vi "Write Test.vi"() -> ()   [LabVIEW 2020]
uses:
  <vilib>/Platform/TimedLoop/XDataNode/timing_clust.ctl
  <vilib>/Platform/TimedLoop/XDataNode/nitl_modes.ctl
  <vilib>/Platform/TimedLoop/XDataNode/wakeup.ctl
  <vilib>/platform/TimedLoop/XDataNode/XDataNode.xnode
  <vilib>/measure/NI_MABase.lvlib
  <vilib>/Platform/TimedLoop/XDataNode/XDNodeRunTimeDep.lvlib
panel:
  out "x-y":dbl
  out "Array":i32[](array[numeric])
  out "x+y":i32[](array[numeric])
  in  "stop":bool
  out "Storage Time":dbl format="%<%H:%M:%S%3u>t"
  in  "Count":i32
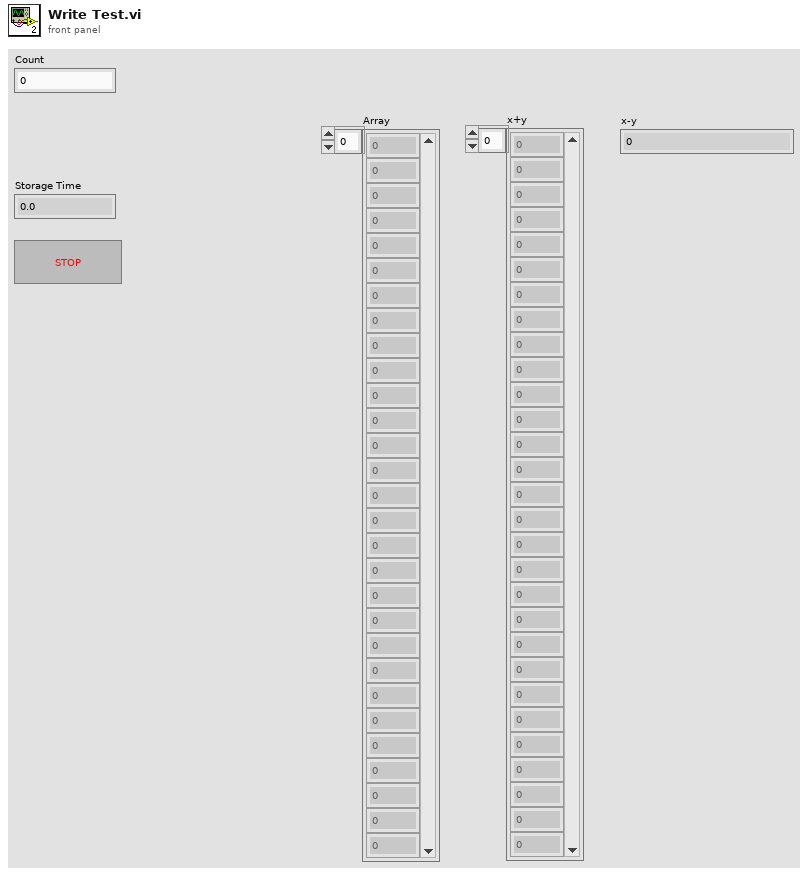
[diagram p1: front panel]
types:
  T1 = enum16{"open", "open or create", "create or replace", "create", "open (read-only)"}
  T2 = typedef "XDNodeRunTimeDep.lvlib/timing_clust.ctl" = cluster{"Expected End [f-1]":u64, "Actual End [f-1]":u64, "Finished Late? [f-1]":bool, "Expected End [i-1]":u64, "Actual End [i-1]":u64, "Finished Late? [i-1]":bool, "Expected Start [i]":u64, "Actual Start [i]":u64, "Expected Start [f]":u64, "Actual Start [f]":u64, "Source Name":string, "Structure Name":string, "Period":i64, "Deadline":i64, "Offset":i64, "Start":i64, "Priority":i32, "Timeout":i32, "Mode":T3, "Wakeup Reason":T4, "Error":errorcluster, "Source Type":string, "Secondary Source Type":string, "Global End Time":u64, "Global Start Time":u64, "Frame Duration":u64, "Iteration Duration":u64, "Assigned CPU":i32, "I/O Scan Engine Mode":u32}
  T3 = typedef "XDNodeRunTimeDep.lvlib/nitl_modes.ctl" = enum32{"No Change", "Process missed periods, maintain original phase", "Discard missed periods, maintain original phase", "Process missed periods, ignore original phase", "Discard missed periods, ignore original phase"}
  T4 = typedef "XDNodeRunTimeDep.lvlib/wakeup.ctl" = enum32{"Normal", "Aborted", "Asynchronous wakeup", "Timing source error", "Timed loop error", "Timeout"}
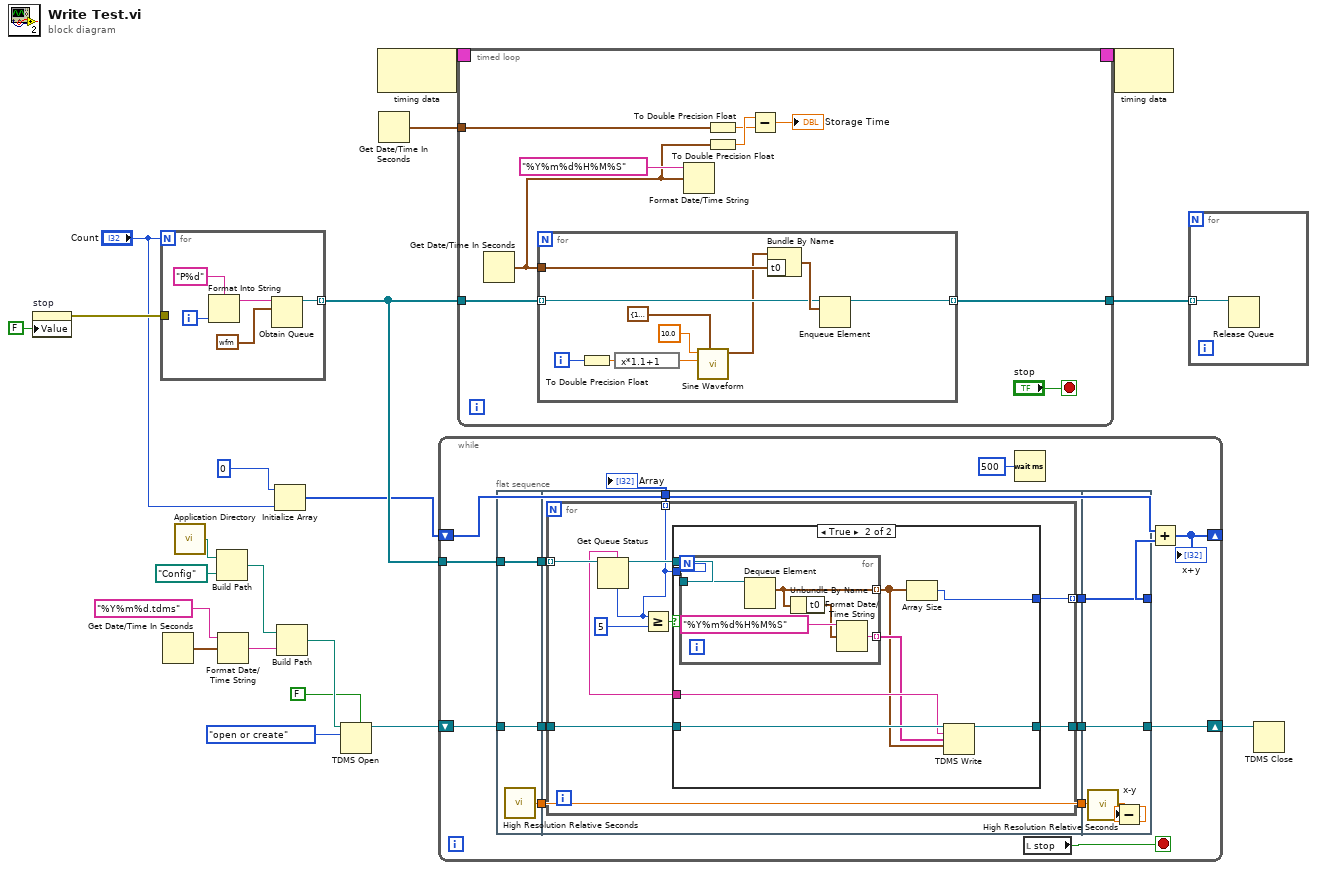
[diagram p0: block diagram]
diagram:
  n1 = property on="stop" class="Bool (strict)"("Value"=FALSE ("stop")) -> (error out=w16:errorcluster)  [unwired: 2 in, 1 out]
  n2 = for {
    N: "Count" -> [_]
    tunnel: [w23] -> w18 mode=indexing
    tunnel: w16 -> [_]
    i -> [w26]
    n3 = Format Into String(format string="P%d", w26) -> (resulting string=w24:string)  [unwired: 2 in, 1 out]
    n4 = Obtain Queue(name (unnamed)=w24, element data type=waveform(dbl) {"t0"=timestamp(0 s since 1904-01-01), "dt"=1.0, "Y"=[]} ("output waveform")) -> (queue out=w23:refnum<queue>)  [unwired: 3 in, 2 out]
  }
  n5 = Get Date/Time In Seconds() -> (seconds since 1Jan1904=w9:timestamp)
  n6 = call <vilib>:"Application Directory.vi"() -> ("Application Directory"=w11:path)
  n7 = Build Path(base path=w11, name or relative path=path "Config") -> (appended path=w8:path)
  n8 = Format Date/Time String(time format string (%c)="%Y%m%d.tdms", seconds (now)=w9) -> (date/time string=w6:string)  [unwired: 1 in]
  n9 = Initialize Array(0, "Count") -> (w12:i32[])
  n10 = Build Path(base path=w8, name or relative path=w6) -> (appended path=w5:path)
  n11 = TDMS Open(5:FALSE ("create index file? (T)"), 10:T1."open or create" ("operation (0:open)"), 11:w5) -> (3:w2:refnum<k34>)  [unwired: 4 in, 1 out]
  n12 = node-c288() -> (w21:T2)  [unwired: 1 in]
  n13 = Get Date/Time In Seconds() -> (seconds since 1Jan1904=w19:timestamp)
  n14 = while {
    tunnel: w18 -> [w41]
    shift-right: [w38] -> _
    shift-left: w12 -> [w37]
    shift-right: [w34] -> w1
    shift-left: w2 -> [w35]
    stop <- w40 stop-if-true
    n15 = flat-sequence {
      tunnel: w35 -> [w43]
      tunnel: w41 -> [w44]
      tunnel: [w44] -> w31
      tunnel: [w43] -> w30
      tunnel: [w42] -> w28
      tunnel: [w48] -> w36
      tunnel: [w49] -> w33
      tunnel: [w46] -> w32
      tunnel: w31 -> [w50]
      tunnel: w30 -> [w47]
      tunnel: [w45] -> w29
      tunnel: w28 -> [w45]
      tunnel: [w77] -> w34
      tunnel: [w78] -> w39
      tunnel: w33 -> [w78]
      tunnel: w32 -> [w77]
      tunnel: w29 -> [w75]
      frame #0 {
        n16 = call <vilib>:"High Resolution Relative Seconds.vi"() -> ("relative seconds"=w42:dbl)
      }
      frame #1 {
        n17 = for {
          tunnel: w50 -> [w59] mode=indexing
          tunnel: [w55] -> w49 mode=indexing
          tunnel: [w54] -> w48 mode=indexing
          tunnel: w47 -> [w53]
          tunnel: [w51] -> w46
          n18 = Get Queue Status(queue=w59) -> (queue out=w58:refnum<queue>, queue name=w52:string, # elements in queue=w54:i32)  [unwired: 2 in, 5 out]
          n19 = Greater Or Equal?(x=w54, y=5) -> (x >= y?=w57:bool)
          n20 = case shown="True" w57 {
            tunnel: w58 -> [_ w67]
            tunnel: [_ w66] -> w55
            tunnel: w54 -> [_ w68]
            tunnel: w53 -> [w60 w65]
            tunnel: w52 -> [_ w64]
            tunnel: [w60 w63] -> w51
            frame False {
            }
            frame True {
              n21 = for {
                N: w68 -> [_]
                tunnel: w67 -> [w73]
                tunnel: [w71] -> w61 mode=indexing
                tunnel: [w69] -> w62 mode=indexing
                n22 = Dequeue Element(queue=w73) -> (element=w71:waveform(dbl))  [unwired: 2 in, 3 out]
                n23 = Unbundle By Name(w71) -> ("t0"=w70:timestamp)
                n24 = Format Date/Time String(time format string (%c)="%Y%m%d%H%M%S", seconds (now)=w70) -> (date/time string=w69:string)  [unwired: 1 in]
              }
              n25 = Array Size(array=w61) -> (size(s)=w66:i32)
              n26 = TDMS Write(0:w65, 5:w64, 7:w62, 9:w61) -> (4:w63:refnum<k34>)  [unwired: 2 in, 3 out]
            }
          }
        }
      }
      frame #2 {
        n27 = call <vilib>:"High Resolution Relative Seconds.vi"() -> ("relative seconds"=w76:dbl)
        n28 = Subtract(x=w76, y=w75) -> (x-y=→"x-y":dbl)
      }
    }
    n29 = Wait (ms)(milliseconds to wait=u32 500) -> ()  [unwired: 1 out]
    n30 = local read "stop"() -> (w40:bool)
    n31 = Add(x=w37, y=w39) -> (x+y=w38:i32[])
    "x+y" <- w38
    "Array" <- w36
  }
  n32 = timed-loop {
    timing: w21 -> [_]
    timing-out: [_] -> w20
    tunnel: w19 -> [w86]
    tunnel: w18 -> [w80]
    tunnel: [w79] -> w17
    stop <- "stop" stop-if-true
    n33 = Get Date/Time In Seconds() -> (seconds since 1Jan1904=w85:timestamp)
    n34 = for {
      tunnel: w85 -> [w92]
      tunnel: w80 -> [w90] mode=indexing
      tunnel: [w88] -> w79 mode=indexing
      i -> [w93]
      n35 = To Double Precision Float(number=w93) -> (double precision float=w94:dbl)
      n36 = expression code="x*1.1+1"(w94) -> (w97:dbl)
      n37 = call <vilib>:"Sine Waveform.vi"("sampling info"=cluster{"Fs":dbl, "#s":dbl} {"Fs"=100.0, "#s"=100.0}, "amplitude"=w97, "frequency"=10.0) -> ("signal out"=w89:waveform(dbl))  [unwired: 7 in, 1 out]
      n38 = Bundle By Name(cluster=w89, "t0"=w92) -> (w91:waveform(dbl))
      n39 = Enqueue Element(queue=w90, element=w91) -> (queue out=w88:refnum<queue>)  [unwired: 2 in, 2 out]
    }
    n40 = Format Date/Time String(time format string (%c)="%Y%m%d%H%M%S", seconds (now)=w85) -> ()  [unwired: 1 in, 1 out]
    n41 = To Double Precision Float(number=w86) -> (double precision float=w83:dbl)
    n42 = To Double Precision Float(number=w85) -> (double precision float=w84:dbl)
    n43 = Subtract(x=w84, y=w83) -> (x-y=→"Storage Time":dbl)
  }
  n44 = node-c288(w20) -> ()  [unwired: 1 out]
  n45 = for {
    tunnel: w17 -> [w100] mode=indexing
    n46 = Release Queue(queue=w100) -> ()  [unwired: 2 in, 3 out]
  }
  n47 = TDMS Close(11:w1) -> ()  [unwired: 1 in, 2 out]
